vi "sabertooth packetized checksum.vi"(1 "Data":u8, 2 "Command":u8, 3 "Address":u8) -> (0 "Checksum":u8)   [LabVIEW 2018]
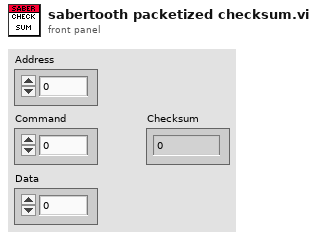
[diagram p1: front panel]
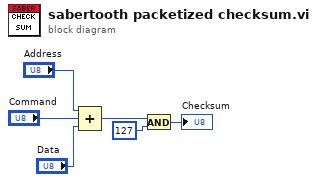
[diagram p0: block diagram]
diagram:
  n1 = Compound Arithmetic op=ADD("Address", "Command", "Data") -> (w3:u8)
  n2 = And(x=w3, y=u8 127) -> (x .and. y?=→"Checksum":u8)
